vi "Parse Response JSON.vi"(8 "error in (no error)":errorcluster, 10 "Response JSON":string, 11 "REmptyResponse in":refnum<class "REmptyResponse.lvclass">) -> (0 "error out":errorcluster, 3 "REmptyResponse out":refnum<class "REmptyResponse.lvclass">)   [LabVIEW 2020, in "obs-websocket.lvlib" / "REmptyResponse.lvclass"]
uses:
  REmptyResponse.lvclass
  REmptyResponse.lvclass/REmptyResponse.ctl
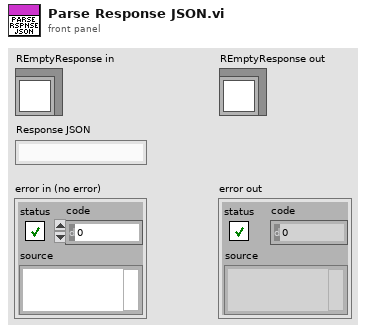
[diagram p1: front panel]
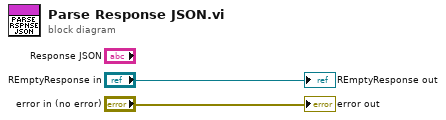
[diagram p0: block diagram]
diagram:
  "error out" <- "error in (no error)"
  "REmptyResponse out" <- "REmptyResponse in"
